vi "Quaternion_GetLVQuat.vi"(11 "Quaternion":T2={"R"=1.0, "V"=[0.0, 0.0, 0.0]}) -> (3 "LV Quaternion":T1)   [LabVIEW 2019, in "Trajectory_Library.lvlib"]
doc: "Convenience constructors that takes in x and y values directly instead of having to construct a Translation2d.\n\nParameters:\n - X- The x component of the translational component of the pose.\n - Y - The y component of the translational component of the pose.\n - Rotation (Heading) - The rotational component of the pose.\n\nReturns:\n - OUT POSE - Output POSE"
uses:
  Trajectory_Library.lvlib
  QUATERNION.ctl
  <vilib>/robotics/Kinematics/Quaternion.ctl
  <vilib>/robotics/Kinematics/NI_Kinematics.lvlib
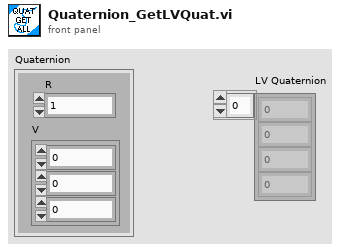
[diagram p1: front panel]
types:
  T1 = typedef "NI_Kinematics.lvlib/Quaternion.ctl" = dbl[]
  T2 = typedef "Trajectory_Library.lvlib/QUATERNION.ctl" = cluster{"R":dbl, "V":dbl[]}
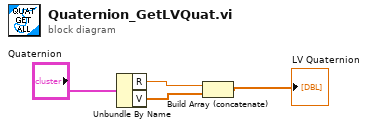
[diagram p0: block diagram]
diagram:
  n1 = Unbundle By Name("Quaternion") -> ("R"=w3:dbl, "V"=w2:dbl[])
  n2 = Build Array (concatenate)(w3, w2) -> (→"LV Quaternion":dbl[])
